vi "Tree Test -2.vi"() -> ()   [LabVIEW 2015]
panel:
  out "number":i32
  out "Single Selection Display Text":string
  in  "Single Selection Tree":string(tree)="Sine Graph"
  in  "Stop":bool
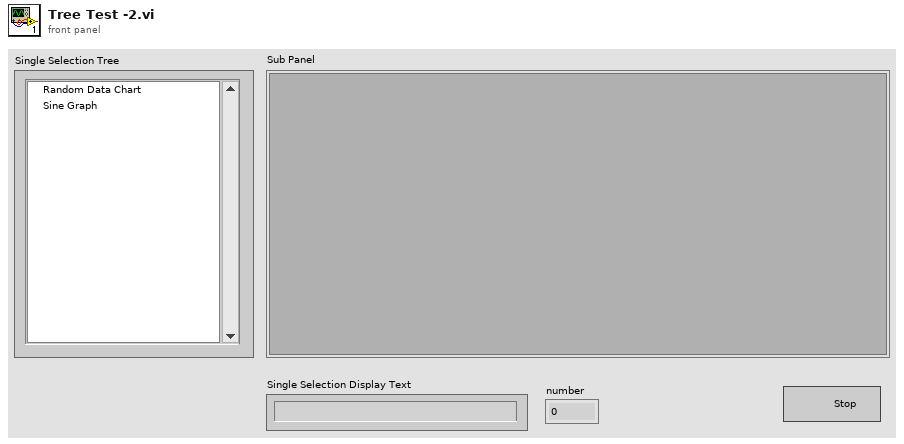
[diagram p1: front panel]
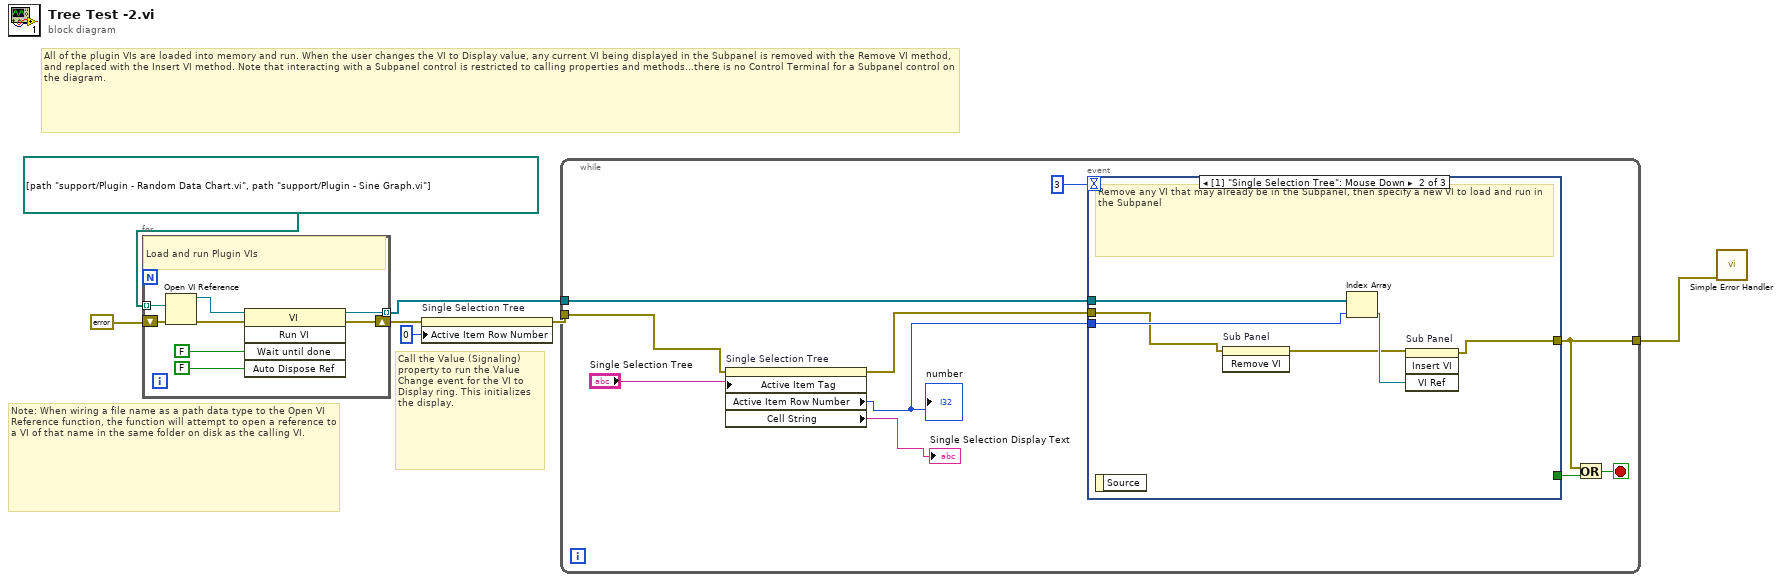
[diagram p0: block diagram]
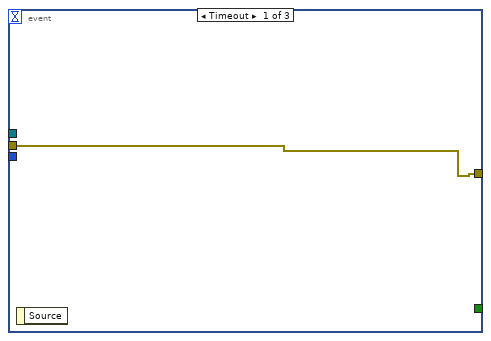
[diagram p2: hidden frame]
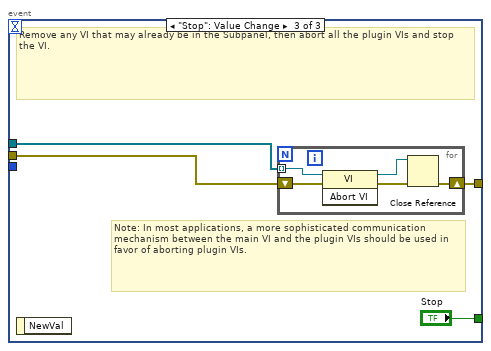
[diagram p3: hidden frame]
diagram:
  # "All of the plugin VIs are loaded into memory and run. When the user changes the VI to Display value, any current VI being displayed in the Subpanel is removed with the Remove VI method, and replaced with the Insert VI method. Note that interacting with a Subpanel control is restricted to calling properties and methods...there is no Control Terminal for a Subpanel control on the diagram."
  # "Note: When wiring a file name as a path data type to the Open VI Reference function, the function will attempt to open a reference to a VI of that name in the same folder on disk as the calling VI."
  # "Call the Value (Signaling) property to run the Value Change event for the VI to Display ring. This initializes the display."
  n1 = for {
    tunnel: path[] [path "support/Plugin - Random Data Chart.vi", path "support/Plugin - Sine Graph.vi"] -> [w11] mode=indexing
    tunnel: [w10] -> w6 mode=indexing
    shift-right: [w8] -> w2
    shift-left: errorcluster {"status"=FALSE, "code"=0, "source"=""} ("error constant") -> [w9]
    # "Load and run Plugin VIs"
    n2 = Open VI Reference(vi path=w11, error in (no error)=w9) -> (vi reference=w12:refnum<vi>, error out=w13:errorcluster)  [unwired: 4 in]
    n3 = invoke class="VI" method="Run VI"(reference=w12, error in=w13, "Wait until done"=FALSE ("Wait Until Done"), "Auto Dispose Ref"=FALSE ("Auto Dispose Reference")) -> (reference out=w10:refnum<vi>, error out=w8:errorcluster)  [unwired: 1 in, 3 out]
  }
  n4 = property on="Single Selection Tree" class="Tree (strict)"(error in=w2, "Active Item Row Number"=0 ("Active Item:Row Number")) -> (error out=w1:errorcluster)  [unwired: 1 in, 1 out]
  n5 = while {
    tunnel: [w23] -> w7
    tunnel: w6 -> [w22]
    tunnel: w1 -> [w18]
    stop <- w24 stop-if-true
    n6 = property on="Single Selection Tree" class="TreeControl (strict)"(error in=w18, "Active Item Tag"="Single Selection Tree") -> (error out=w17:errorcluster, "Active Item Row Number"=w16:i32, "Cell String"=→"Single Selection Display Text":string)  [unwired: 1 in, 1 out]
    "number" <- w16
    n7 = event shown="[1] \"Single Selection Tree\": Mouse Down" {
      selector: _ -> [_ _ _]
      dyn-events: _ -> [_ _ _]
      timeout: 3 -> [_ _ _]
      tunnel: [_ _ "Stop"] -> w25
      tunnel: [w26 w30 w34] -> w23
      tunnel: w22 -> [_ w32 w35]
      tunnel: w17 -> [w26 w27 w33]
      tunnel: w16 -> [_ w28 _]
      event Timeout {
        n8 = event-data() -> ()  [unwired: 1 in, 1 out]
      }
      event "Single Selection Tree": Mouse Down {
        # "Remove any VI that may already be in the Subpanel, then specify a new VI to load and run in the Subpanel"
        n9 = event-data() -> ()  [unwired: 1 in, 1 out]
        n10 = invoke on="Sub Panel" class="SubPnl" method="Remove VI"(error in=w27) -> (error out=w29:errorcluster)  [unwired: 2 in, 2 out]
        n11 = Index Array(array=w32, index=w28) -> (element=w31:refnum<vi>)
        n12 = invoke on="Sub Panel" class="SubPnl" method="Insert VI"(error in=w29, "VI Ref"=w31) -> (error out=w30:errorcluster)  [unwired: 2 in, 3 out]
      }
      event "Stop": Value Change {
        # "Note: In most applications, a more sophisticated communication mechanism between the main VI and the plugin VIs should be used in favor of aborting plugin VIs."
        # "Remove any VI that may already be in the Subpanel, then abort all the plugin VIs and stop the VI."
        n13 = event-data() -> ()  [unwired: 1 in, 1 out]
        n14 = for {
          shift-right: [w37] -> w34
          shift-left: w33 -> [w41]
          tunnel: w35 -> [w40] mode=indexing
          n15 = invoke class="VI" method="Abort VI"(reference=w40, error in=w41) -> (reference out=w38:refnum<vi>, error out=w39:errorcluster)  [unwired: 1 in, 1 out]
          n16 = Close Reference(reference=w38, error in (no error)=w39) -> (error out=w37:errorcluster)
        }
      }
    }
    n17 = Or(x=w23, y=w25) -> (x .or. y?=w24:bool)
  }
  n18 = call <vilib>:"Simple Error Handler.vi"("error in (no error)"=w7) -> ()  [unwired: 4 in, 5 out]
